vi "TakeMeasAtSomeFrequency.vi"(7 "Generator Frequency":dbl, 8 "GEN error":errorcluster, 9 "GEN VISA":refnum<visa-resource-name>, 10 "Scope Error":errorcluster, 11 "Scope VISA":refnum<visa-resource-name>) -> (0 "GEN Error OUT":errorcluster, 1 "GEN VISA OUT":refnum<visa-resource-name>, 2 "Scope error out":errorcluster, 3 "Scope VISA out":refnum<visa-resource-name>, 4 "max value":dbl, 6 "dt":dbl)   [LabVIEW 2021]
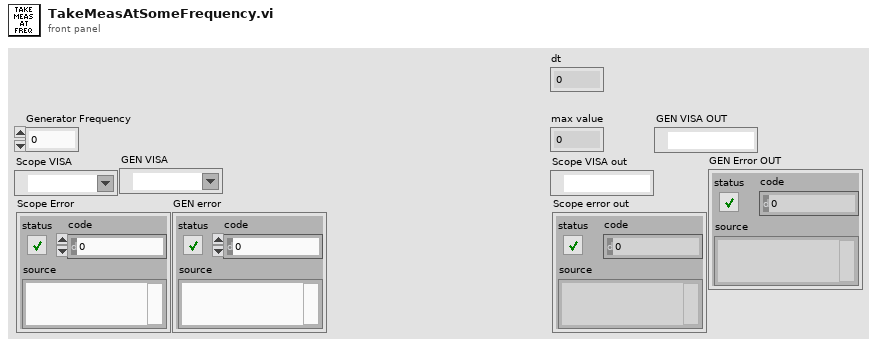
[diagram p1: front panel]
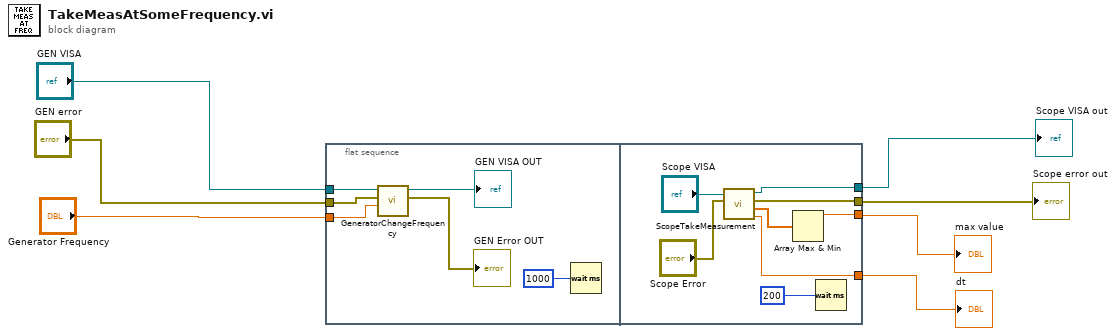
[diagram p0: block diagram]
diagram:
  n1 = flat-sequence {
    tunnel: "Generator Frequency" -> [w12]
    tunnel: "GEN VISA" -> [w11]
    tunnel: "GEN error" -> [w10]
    tunnel: [w18] -> w6
    tunnel: [w17] -> w4
    tunnel: [w16] -> w5
    tunnel: [w15] -> w1
    frame #0 {
      n2 = call "GeneratorChangeFrequency.vi"("GeneratorChangeFreq"=w12, "GEN error"=w10, "GEN VISA"=w11) -> ("error out"=→"GEN Error OUT":errorcluster, "VISA resource name out"=→"GEN VISA OUT":refnum<visa-resource-name>)  [unwired: 7 in]
      n3 = Wait (ms)(milliseconds to wait=u32 1000) -> ()  [unwired: 1 out]
    }
    frame #1 {
      n4 = call "ScopeTakeMeasurement.vi"("Scope Error"="Scope Error", "Scope VISA"="Scope VISA") -> ("dt"=w15:dbl, "Data"=w19:dbl[], "error out"=w17:errorcluster, "VISA resource name out"=w16:refnum<visa-resource-name>)  [unwired: 6 in]
      n5 = Array Max & Min(array=w19) -> (max value=w18:dbl)  [unwired: 3 out]
      n6 = Wait (ms)(milliseconds to wait=u32 200) -> ()  [unwired: 1 out]
    }
  }
  "max value" <- w6
  "Scope VISA out" <- w5
  "Scope error out" <- w4
  "dt" <- w1
